vi "initialize redirection.vi"(11 "Oauth2":refnum<class "Oauth2.lvclass">) -> (3 "Redirect URI":refnum<class "URI.lvclass">)   [LabVIEW 2013, in "Oauth2.lvclass"]
uses:
  Oauth2.lvclass
  <vilib>/LabVIEW Open Source Project/OpenURI/uri/URI.lvclass
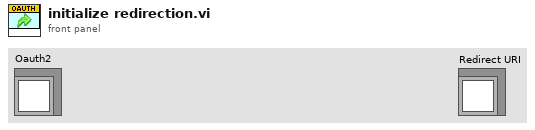
[diagram p1: front panel]
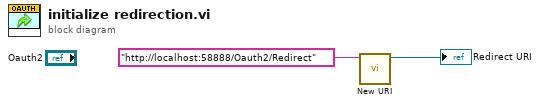
[diagram p0: block diagram]
diagram:
  n1 = call <vilib>:"New URI.vi"("URI"="http://localhost:58888/Oauth2/Redirect") -> ("URI"=→"Redirect URI":refnum<class "URI.lvclass">)  [unwired: 9 in, 1 out]
